vi "Page_Exclusions_Initialize.vi"(8 "error in (no error)":errorcluster, 9 "ctlReferences":T1, 11 "AB_Build in":refnum<class "AB_Build.lvclass">) -> (0 "error out":errorcluster, 3 "AB_Build out":refnum<class "AB_Build.lvclass">)   [LabVIEW 2020, in "AB_Build.lvclass"]
uses:
  <vilib>/AppBuilder/AB_Classes/Build/AB_Build.lvclass
  <resource>/Framework/Providers/Builds/AppBuilder/AB_UI_Page_Exclusions_References.ctl
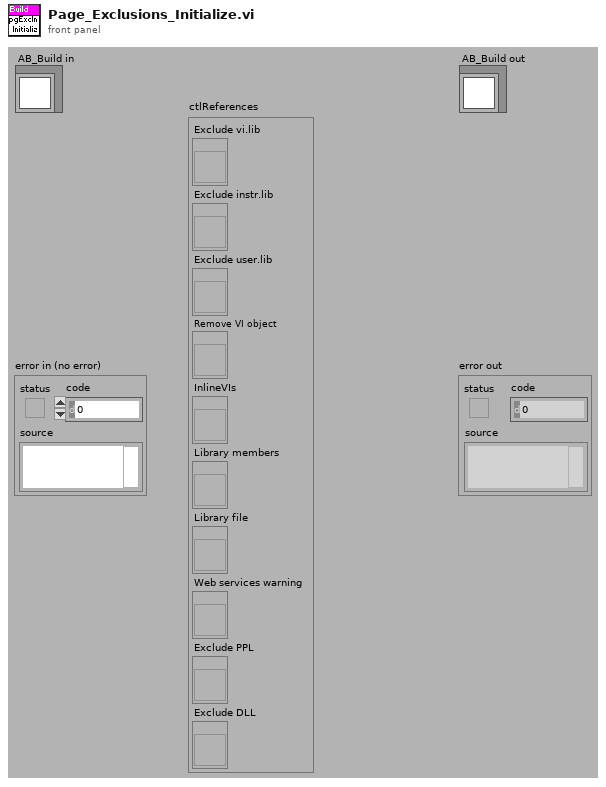
[diagram p1: front panel]
types:
  T1 = typedef "AB_UI_Page_Exclusions_References.ctl" = cluster{"Exclude vi.lib":refnum<vi>, "Exclude instr.lib":refnum<vi>, "Exclude user.lib":refnum<vi>, "Remove VI object":refnum<vi>, "InlineVIs":refnum<vi>, "Library members":refnum<vi>, "Library file":refnum<vi>, "Web services warning":refnum<vi>, "Exclude PPL":refnum<vi>, "Exclude DLL":refnum<vi>}
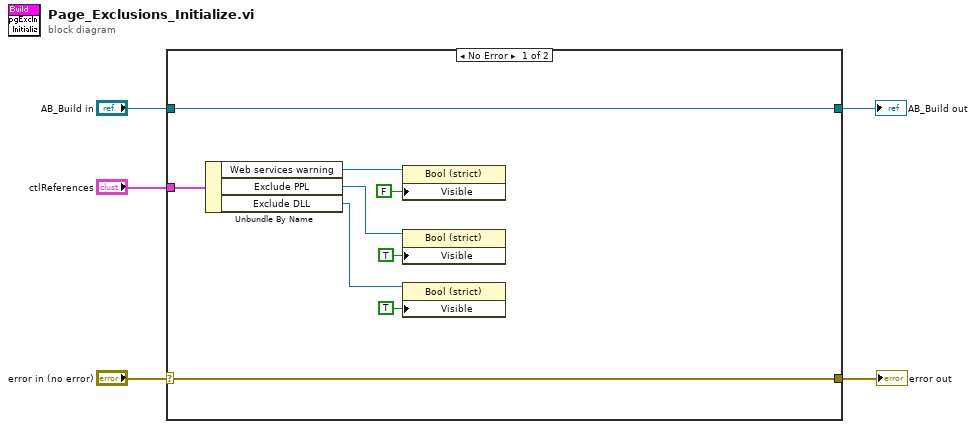
[diagram p0: block diagram]
diagram:
  n1 = case shown="No Error" "error in (no error)" {
    selector: "error in (no error)" -> [w13 w16]
    tunnel: [w13 w16] -> w4
    tunnel: [w14 w15] -> w2
    tunnel: "AB_Build in" -> [w14 w15]
    tunnel: "ctlReferences" -> [w12 _]
    frame No Error {
      n2 = Unbundle By Name(w12) -> ("Web services warning"=w11:refnum<vi>, "Exclude PPL"=w8:refnum<vi>, "Exclude DLL"=w6:refnum<vi>)
      n3 = property class="Bool (strict)"(reference=w11, "Visible"=FALSE) -> ()  [unwired: 1 in, 2 out]
      n4 = property class="Bool (strict)"(reference=w8, "Visible"=TRUE) -> ()  [unwired: 1 in, 2 out]
      n5 = property class="Bool (strict)"(reference=w6, "Visible"=TRUE) -> ()  [unwired: 1 in, 2 out]
    }
    frame Error {
    }
  }
  "error out" <- w4
  "AB_Build out" <- w2
